vi "Load Measurements from Disk.vi"(8 "error in (no error)":errorcluster, 10 "Array of paths (folders to scan or explicit files)":path[](array[path]), 11 "base path":path) -> (0 "error out":errorcluster, 2 "Available Measurements":refnum<class "Measurement.lvclass">[](array[class]))   [LabVIEW 2017, in "Controller Actor.lvlib" / "Controller.lvclass"]
uses:
  Controller.lvclass
  Measurement Actor/Measurement.lvclass
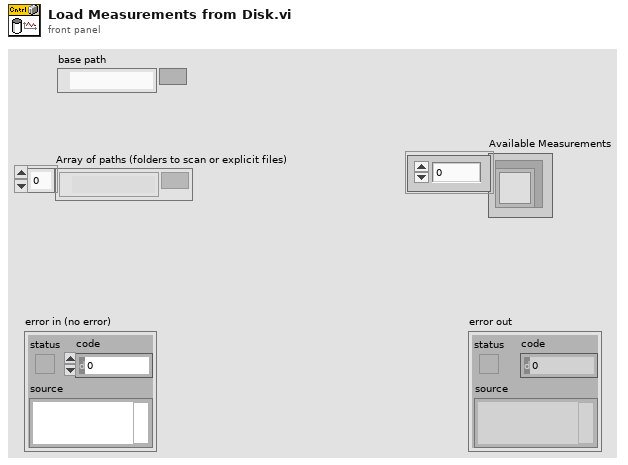
[diagram p1: front panel]
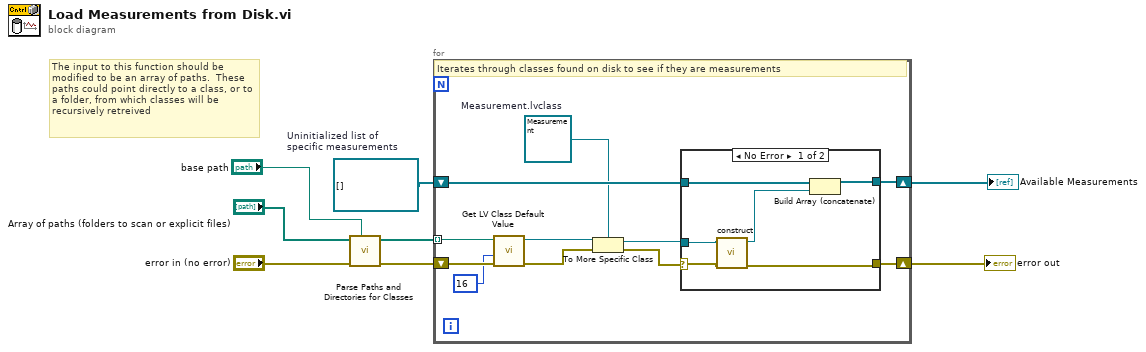
[diagram p0: block diagram]
diagram:
  w8 = refnum<class "Measurement.lvclass">[] []  # Uninitialized list of specific measurements
  # "The input to this function should be modified to be an array of paths.  These paths could point directly to a class, or to a folder, from which classes will be recursively retreived"
  n1 = call "Parse Paths and Directories for Classes.vi"("base path"="base path", "error in (no error)"="error in (no error)", "Array of paths (folders to scan or explicit files)"="Array of paths (folders to scan or explicit files)") -> ("error out"=w4:errorcluster, "All Files in Dir"=w5:path[])  [unwired: 7 in]
  n2 = for {
    shift-right: [w18] -> w7
    shift-left: w8 -> [w14]
    shift-right: [w15] -> w6
    shift-left: w4 -> [w16]
    tunnel: w5 -> [w9] mode=indexing
    w12 = refnum<class "Measurement.lvclass"> refnum  # Measurement.lvclass
    # "Iterates through classes found on disk to see if they are measurements"
    n3 = call <vilib>:"Get LV Class Default Value.vi"("error in (no error)"=w16, "options"=u32 16, "class path"=w9) -> ("error out"=w17:errorcluster, "object"=w13:refnum<class>)  [unwired: 7 in]
    n4 = To More Specific Class(target class=w12, reference=w13, error in=w17) -> (specific class reference=w19:refnum<class "Measurement.lvclass">, error out=w11:errorcluster)
    n5 = case shown="No Error" w11 {
      selector: w11 -> [w22 _]
      tunnel: w19 -> [w23 _]
      tunnel: [w25 w26] -> w18
      tunnel: w14 -> [w24 w26]
      tunnel: [w20 _] -> w15
      frame No Error {
        n6 = call-dynamic "construct.vi"("error in (no error)"=w22, "Measurement in"=w23) -> ("error out"=w20:errorcluster, "Measurement out"=w21:refnum<class "Measurement.lvclass">)  [unwired: 8 in]
        n7 = Build Array (concatenate)(w24, w21) -> (w25:refnum<class "Measurement.lvclass">[])
      }
      frame Error {
      }
    }
  }
  "error out" <- w6
  "Available Measurements" <- w7
